vi "update.vi"(8 "error in (no error)":errorcluster, 11 "FPGAWrapperDL120115Galvo in":refnum<class "FPGAWrapperDL090211Galvo.lvclass">) -> (0 "error out":errorcluster, 3 "FPGAWrapperDL120115Galvo out":refnum<class "FPGAWrapperDL090211Galvo.lvclass">)   [LabVIEW 2010, in "FPGAWrapperDL090211Galvo.lvclass"]
uses:
  FPGAWrapperDL090211Galvo.lvclass
  type definitions/command_enum.ctl
  FPGAWrapperDL090211Galvo.lvclass/FPGAWrapperDL090211Galvo.ctl
  class_data.vi
panel:
  out "number of pixels":i64
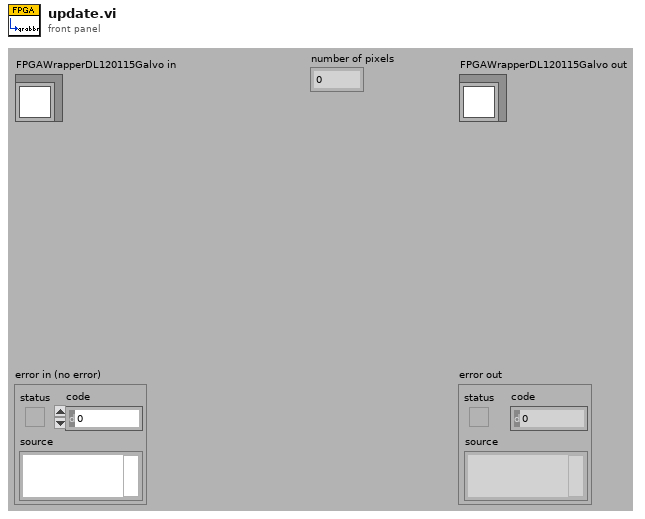
[diagram p1: front panel]
types:
  T1 = typedef "command_enum.ctl" = enum16{"NULL", "update", "start", "stop", "reset", "shut-down"}
  T2 = typedef "settings_cluster.ctl" = cluster{"number of pixels":i64, "pixel frequency (Hz)":dbl, "pixel values cluster":T3, "triggered?":bool, "triggered flag valid?":bool, "gates":T4[]}
  T3 = typedef "channels_cluster.ctl" = cluster{"channel 0":u32, "channel 1":u32, "channel 2":u32, "channel 3":u32}
  T4 = typedef "gate_cluster.ctl" = cluster{"index":i32, "parameters":T5}
  T5 = typedef "gate_parameters_cluster.ctl" = cluster{"offset":i64, "pulsing":i64, "not pulsing":i64, "cycles per pulse":i64, "repetitions":i64}
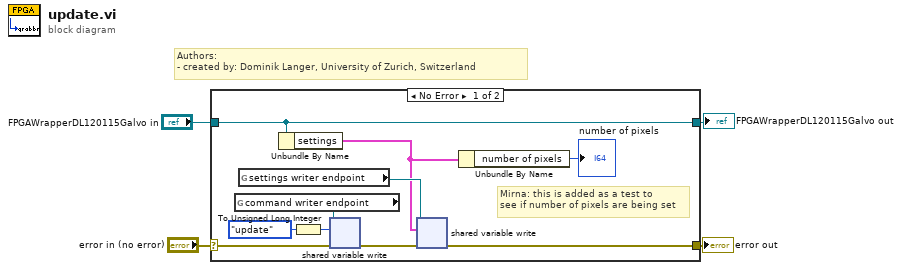
[diagram p0: block diagram]
diagram:
  # "Authors: \n- created by: Dominik Langer, University of Zurich, Switzerland"
  n1 = case shown="No Error" "error in (no error)" {
    selector: "error in (no error)" -> [w11 w16]
    tunnel: [w9 w16] -> w3
    tunnel: [w12 w15] -> w1
    tunnel: "FPGAWrapperDL120115Galvo in" -> [w12 w15]
    frame No Error {
      # "Mirna: this is added as a test to \nsee if number of pixels are being set"
      n2 = global read "class_data.vi" "command writer endpoint"() -> (w8:refnum<k21>)
      n3 = global read "class_data.vi" "settings writer endpoint"() -> (w7:refnum<k21>)
      n4 = Unbundle By Name(w12) -> ("settings"=w6:T2)
      n5 = To Unsigned Long Integer(number=command_enum."update" ("command")) -> (unsigned 32bit integer=w14:u32)
      n6 = shared-variable-write(w8, w11, w14) -> (w10:errorcluster)  [unwired: 1 in, 2 out]
      n7 = shared-variable-write(w7, w10, w6) -> (w9:errorcluster)  [unwired: 1 in, 2 out]
      n8 = Unbundle By Name(w6) -> ("number of pixels"=→"number of pixels":i64)
    }
    frame Error {
    }
  }
  "error out" <- w3
  "FPGAWrapperDL120115Galvo out" <- w1
